vi "PlayMusic.vi"(0 "reference in":refnum<class "MediaPlayer.lvclass">, 11 "Error In":errorcluster) -> (4 "reference out":refnum<class "MediaPlayer.lvclass">, 15 "Error Out":errorcluster)   [LabVIEW 2024, in "MediaPlayer.lvclass"]
doc: "Starts playing current Song Handled music"
uses:
  MediaPlayer.lvclass
  MediaPlayer.lvclass/MediaPlayer.ctl
panel:
  # "Connector Pane"
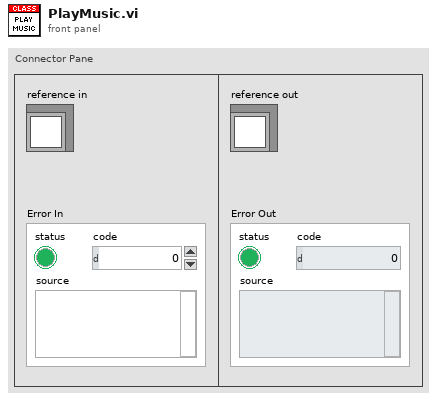
[diagram p1: front panel]
types:
  T1 = typedef "MediaPlayer.lvclass/ObjectAttributes.ctl" = cluster{"MediaPlayerData":T2, "Current Info":T4}
  T2 = typedef "MediaPlayer.lvclass/MediaPlayer Data.ctl" = cluster{"Music List":path[], "Current Music Index":i64, "Song Handler":T3, "Device ID":u32}
  T3 = typedef "Sound Output Task ID.ctl" = u32
  T4 = typedef "MediaPlayer.lvclass/Current Info.ctl" = cluster{"Duration":dbl, "Name":string, "Is playing?":bool, "Current Music Index":i64}
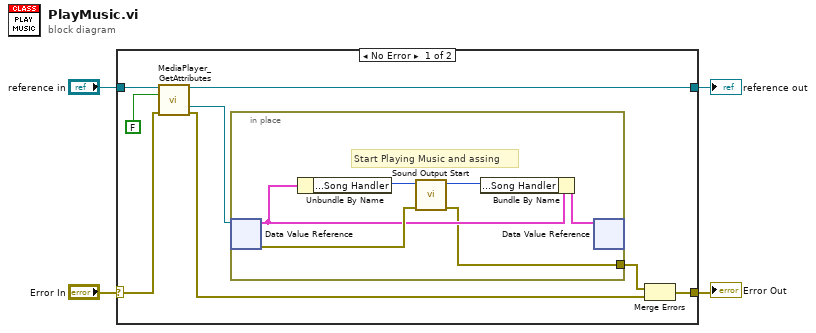
[diagram p0: block diagram]
diagram:
  n1 = case shown="No Error" "Error In" {
    selector: "Error In" -> [w11 w20]
    tunnel: [w6 w20] -> w3
    tunnel: [w10 w19] -> w1
    tunnel: "reference in" -> [w12 w19]
    frame No Error {
      n2 = call "MediaPlayer_GetAttributes.vi"("reference in"=w12, "OnlyGetDvrReference(False)"=FALSE, "Error In"=w11) -> ("reference out"=w10:refnum<class "MediaPlayer.lvclass">, "DataRef"=w7:refnum<data-value>, "Error Out"=w8:errorcluster)  [unwired: 9 in, 1 out]
      n3 = in-place {
        in-place-border: [w15] -> w5
        # "Start Playing Music and assing"
        n4 = in-place-dvr #1(w7) -> (w16:T1, w17:errorcluster)
        n5 = Unbundle By Name(w16) -> ("MediaPlayerData.Song Handler"=w18:T3)
        n6 = call <vilib>:"Sound Output Start.vi"("error in (no error)"=w17, "task ID"=w18) -> ("error out"=w15:errorcluster, "task ID out"=w13:T3)  [unwired: 8 in]
        n7 = Bundle By Name(cluster=w16, "MediaPlayerData.Song Handler"=w13) -> (w14:T1)
        n8 = in-place-dvr #1(w14) -> ()  [unwired: 2 out]
      }
      n9 = Merge Errors(w5, w8) -> (w6:errorcluster)
    }
    frame Error {
    }
  }
  "Error Out" <- w3
  "reference out" <- w1
